vi "LCR_SelectiveWriter.vi"(8 "error in (no error)":errorcluster, 9 "Data Cluster":T3, 10 "Configuration Cluster":T1={"General"={"Config.ini"=path "", "Default Logging Path"=path ""}, "Hardware"={"LCR VISA COM"="", "Measure Rate (1/s)"=0, "Reset on Load?"=FALSE, "Measure Profile"=path ""}, "HM8118 Current Profile"={"Bias Profile"={" Bias Source (OFF)"=0, " Bias Type (Voltage)"=0, "Bias Level (0)"=0.0}, "Measurement Profile"={"Operation Mode (0: Auto)"=0, "Circuit Type (2: Auto)"=2, "Manual Range (1:Range 1 and 25 Ohms)"=1, "Auto Range (T: Enable)"=TRUE}, "Signal Profile"={"Frequency (1kHz)"=1000.0, "Measuring Voltage (1V)"=1.0}, "Integration Profile"={"Averaging (0: Off)"=0, "Averaging Number (2)"=2, "Time (100ms)"=100, "Rate (0: Fast)"=0}, "Trigger Profile"={"Trigger Mode (0: Continuous)"=0}}, "HM8118 New Profile"={"Bias Profile"={" Bias Source (OFF)"=0, " Bias Type (Voltage)"=0, "Bias Level (0)"=0.0}, "Measurement Profile"={"Operation Mode (0: Auto)"=0, "Circuit Type (2: Auto)"=2, "Manual Range (1:Range 1 and 25 Ohms)"=1, "Auto Range (T: Enable)"=TRUE}, "Signal Profile"={"Frequency (1kHz)"=1000.0, "Measuring Voltage (1V)"=1.0}, "Integration Profile"={"Averaging (0: Off)"=0, "Averaging Number (2)"=2, "Time (100ms)"=100, "Rate (0: Fast)"=0}, "Trigger Profile"={"Trigger Mode (0: Continuous)"=0}}, "Operation"={"Operation Mode"=enum."Logging"}} {"HM8118 New Profile"."Trigger Profile"."Trigger Mode (0: Continuous)" items=["Continuous", "Manual", "External"]; "HM8118 New Profile"."Integration Profile"."Rate (0: Fast)" items=["Fast", "Medium", "Slow"]; "HM8118 New Profile"."Integration Profile"."Time (100ms)" min=1 max=999; "HM8118 New Profile"."Integration Profile"."Averaging Number (2)" min=2 max=99; "HM8118 New Profile"."Integration Profile"."Averaging (0: Off)" items=["Off", "Normal", "Averaging"]; "HM8118 New Profile"."Signal Profile"."Measuring Voltage (1V)" min=0.05 max=1.5 step=0.01; "HM8118 New Profile"."Signal Profile"."Frequency (1kHz)" min=20.0 max=200000.0; "HM8118 New Profile"."Measurement Profile"."Manual Range (1:Range 1 and 25 Ohms)" items=["Range 1 and 25 Ohms"=1, "Range 2 and 25 Ohms"=2, "Range 3 and 400 Ohms"=3, "Range 4 and 6.4 kOhms"=4, "Range 5 and 100kOhms"=5, "Range 6 and 100kOhms"=6]; "HM8118 New Profile"."Measurement Profile"."Circuit Type (2: Auto)" items=["Series", "Parallel", "Auto"]; "HM8118 New Profile"."Measurement Profile"."Operation Mode (0: Auto)" items=["Auto", "L+Q", "L+R", "C+D", "C+R", "R+Q", "Z+Theta", "Y+Theta", "R+X", "G+B", "N+Theta", "M"]; "HM8118 New Profile"."Bias Profile"."Bias Type (Voltage)" items=["Voltage", "Current"]; "HM8118 New Profile"."Bias Profile"."Bias Source (OFF)" items=["Off", "Internal", "External"]; "HM8118 Current Profile"."Trigger Profile"."Trigger Mode (0: Continuous)" items=["Continuous", "Manual", "External"]; "HM8118 Current Profile"."Integration Profile"."Rate (0: Fast)" items=["Fast", "Medium", "Slow"]; "HM8118 Current Profile"."Integration Profile"."Time (100ms)" min=1 max=999; "HM8118 Current Profile"."Integration Profile"."Averaging Number (2)" min=2 max=99; "HM8118 Current Profile"."Integration Profile"."Averaging (0: Off)" items=["Off", "Normal", "Averaging"]; "HM8118 Current Profile"."Signal Profile"."Measuring Voltage (1V)" min=0.05 max=1.5 step=0.01; "HM8118 Current Profile"."Signal Profile"."Frequency (1kHz)" min=20.0 max=200000.0; "HM8118 Current Profile"."Measurement Profile"."Manual Range (1:Range 1 and 25 Ohms)" items=["Range 1 and 25 Ohms"=1, "Range 2 and 25 Ohms"=2, "Range 3 and 400 Ohms"=3, "Range 4 and 6.4 kOhms"=4, "Range 5 and 100kOhms"=5, "Range 6 and 100kOhms"=6]; "HM8118 Current Profile"."Measurement Profile"."Circuit Type (2: Auto)" items=["Series", "Parallel", "Auto"]; "HM8118 Current Profile"."Measurement Profile"."Operation Mode (0: Auto)" items=["Auto", "L+Q", "L+R", "C+D", "C+R", "R+Q", "Z+Theta", "Y+Theta", "R+X", "G+B", "N+Theta", "M"]; "HM8118 Current Profile"."Bias Profile"."Bias Type (Voltage)" items=["Voltage", "Current"]; "HM8118 Current Profile"."Bias Profile"."Bias Source (OFF)" items=["Off", "Internal", "External"]}) -> (0 "error out":errorcluster, 2 "Configuration Cluster Out":T1={"General"={"Config.ini"=path "", "Default Logging Path"=path ""}, "Hardware"={"LCR VISA COM"="", "Measure Rate (1/s)"=0, "Reset on Load?"=FALSE, "Measure Profile"=path ""}, "HM8118 Current Profile"={"Bias Profile"={" Bias Source (OFF)"=0, " Bias Type (Voltage)"=0, "Bias Level (0)"=0.0}, "Measurement Profile"={"Operation Mode (0: Auto)"=0, "Circuit Type (2: Auto)"=2, "Manual Range (1:Range 1 and 25 Ohms)"=1, "Auto Range (T: Enable)"=TRUE}, "Signal Profile"={"Frequency (1kHz)"=1000.0, "Measuring Voltage (1V)"=1.0}, "Integration Profile"={"Averaging (0: Off)"=0, "Averaging Number (2)"=2, "Time (100ms)"=100, "Rate (0: Fast)"=0}, "Trigger Profile"={"Trigger Mode (0: Continuous)"=0}}, "HM8118 New Profile"={"Bias Profile"={" Bias Source (OFF)"=0, " Bias Type (Voltage)"=0, "Bias Level (0)"=0.0}, "Measurement Profile"={"Operation Mode (0: Auto)"=0, "Circuit Type (2: Auto)"=2, "Manual Range (1:Range 1 and 25 Ohms)"=1, "Auto Range (T: Enable)"=TRUE}, "Signal Profile"={"Frequency (1kHz)"=1000.0, "Measuring Voltage (1V)"=1.0}, "Integration Profile"={"Averaging (0: Off)"=0, "Averaging Number (2)"=2, "Time (100ms)"=100, "Rate (0: Fast)"=0}, "Trigger Profile"={"Trigger Mode (0: Continuous)"=0}}, "Operation"={"Operation Mode"=enum."Logging"}} {"HM8118 New Profile"."Trigger Profile"."Trigger Mode (0: Continuous)" items=["Continuous", "Manual", "External"]; "HM8118 New Profile"."Integration Profile"."Rate (0: Fast)" items=["Fast", "Medium", "Slow"]; "HM8118 New Profile"."Integration Profile"."Time (100ms)" min=1 max=999; "HM8118 New Profile"."Integration Profile"."Averaging Number (2)" min=2 max=99; "HM8118 New Profile"."Integration Profile"."Averaging (0: Off)" items=["Off", "Normal", "Averaging"]; "HM8118 New Profile"."Signal Profile"."Measuring Voltage (1V)" min=0.05 max=1.5 step=0.01; "HM8118 New Profile"."Signal Profile"."Frequency (1kHz)" min=20.0 max=200000.0; "HM8118 New Profile"."Measurement Profile"."Manual Range (1:Range 1 and 25 Ohms)" items=["Range 1 and 25 Ohms"=1, "Range 2 and 25 Ohms"=2, "Range 3 and 400 Ohms"=3, "Range 4 and 6.4 kOhms"=4, "Range 5 and 100kOhms"=5, "Range 6 and 100kOhms"=6]; "HM8118 New Profile"."Measurement Profile"."Circuit Type (2: Auto)" items=["Series", "Parallel", "Auto"]; "HM8118 New Profile"."Measurement Profile"."Operation Mode (0: Auto)" items=["Auto", "L+Q", "L+R", "C+D", "C+R", "R+Q", "Z+Theta", "Y+Theta", "R+X", "G+B", "N+Theta", "M"]; "HM8118 New Profile"."Bias Profile"."Bias Type (Voltage)" items=["Voltage", "Current"]; "HM8118 New Profile"."Bias Profile"."Bias Source (OFF)" items=["Off", "Internal", "External"]; "HM8118 Current Profile"."Trigger Profile"."Trigger Mode (0: Continuous)" items=["Continuous", "Manual", "External"]; "HM8118 Current Profile"."Integration Profile"."Rate (0: Fast)" items=["Fast", "Medium", "Slow"]; "HM8118 Current Profile"."Integration Profile"."Time (100ms)" min=1 max=999; "HM8118 Current Profile"."Integration Profile"."Averaging Number (2)" min=2 max=99; "HM8118 Current Profile"."Integration Profile"."Averaging (0: Off)" items=["Off", "Normal", "Averaging"]; "HM8118 Current Profile"."Signal Profile"."Measuring Voltage (1V)" min=0.05 max=1.5 step=0.01; "HM8118 Current Profile"."Signal Profile"."Frequency (1kHz)" min=20.0 max=200000.0; "HM8118 Current Profile"."Measurement Profile"."Manual Range (1:Range 1 and 25 Ohms)" items=["Range 1 and 25 Ohms"=1, "Range 2 and 25 Ohms"=2, "Range 3 and 400 Ohms"=3, "Range 4 and 6.4 kOhms"=4, "Range 5 and 100kOhms"=5, "Range 6 and 100kOhms"=6]; "HM8118 Current Profile"."Measurement Profile"."Circuit Type (2: Auto)" items=["Series", "Parallel", "Auto"]; "HM8118 Current Profile"."Measurement Profile"."Operation Mode (0: Auto)" items=["Auto", "L+Q", "L+R", "C+D", "C+R", "R+Q", "Z+Theta", "Y+Theta", "R+X", "G+B", "N+Theta", "M"]; "HM8118 Current Profile"."Bias Profile"."Bias Type (Voltage)" items=["Voltage", "Current"]; "HM8118 Current Profile"."Bias Profile"."Bias Source (OFF)" items=["Off", "Internal", "External"]})   [LabVIEW 2021]
uses:
  Config_Cluster.ctl
  Mode_Enum.ctl
  Data_Cluster.ctl
  Measurement_Cluster.ctl
  LCR_WriteBias.vi
  LCR_WriteConfigMeas.vi
  LCR_WriteSignal.vi
  LCR_WriteIntegration.vi
  LCR_WriteTrigger.vi
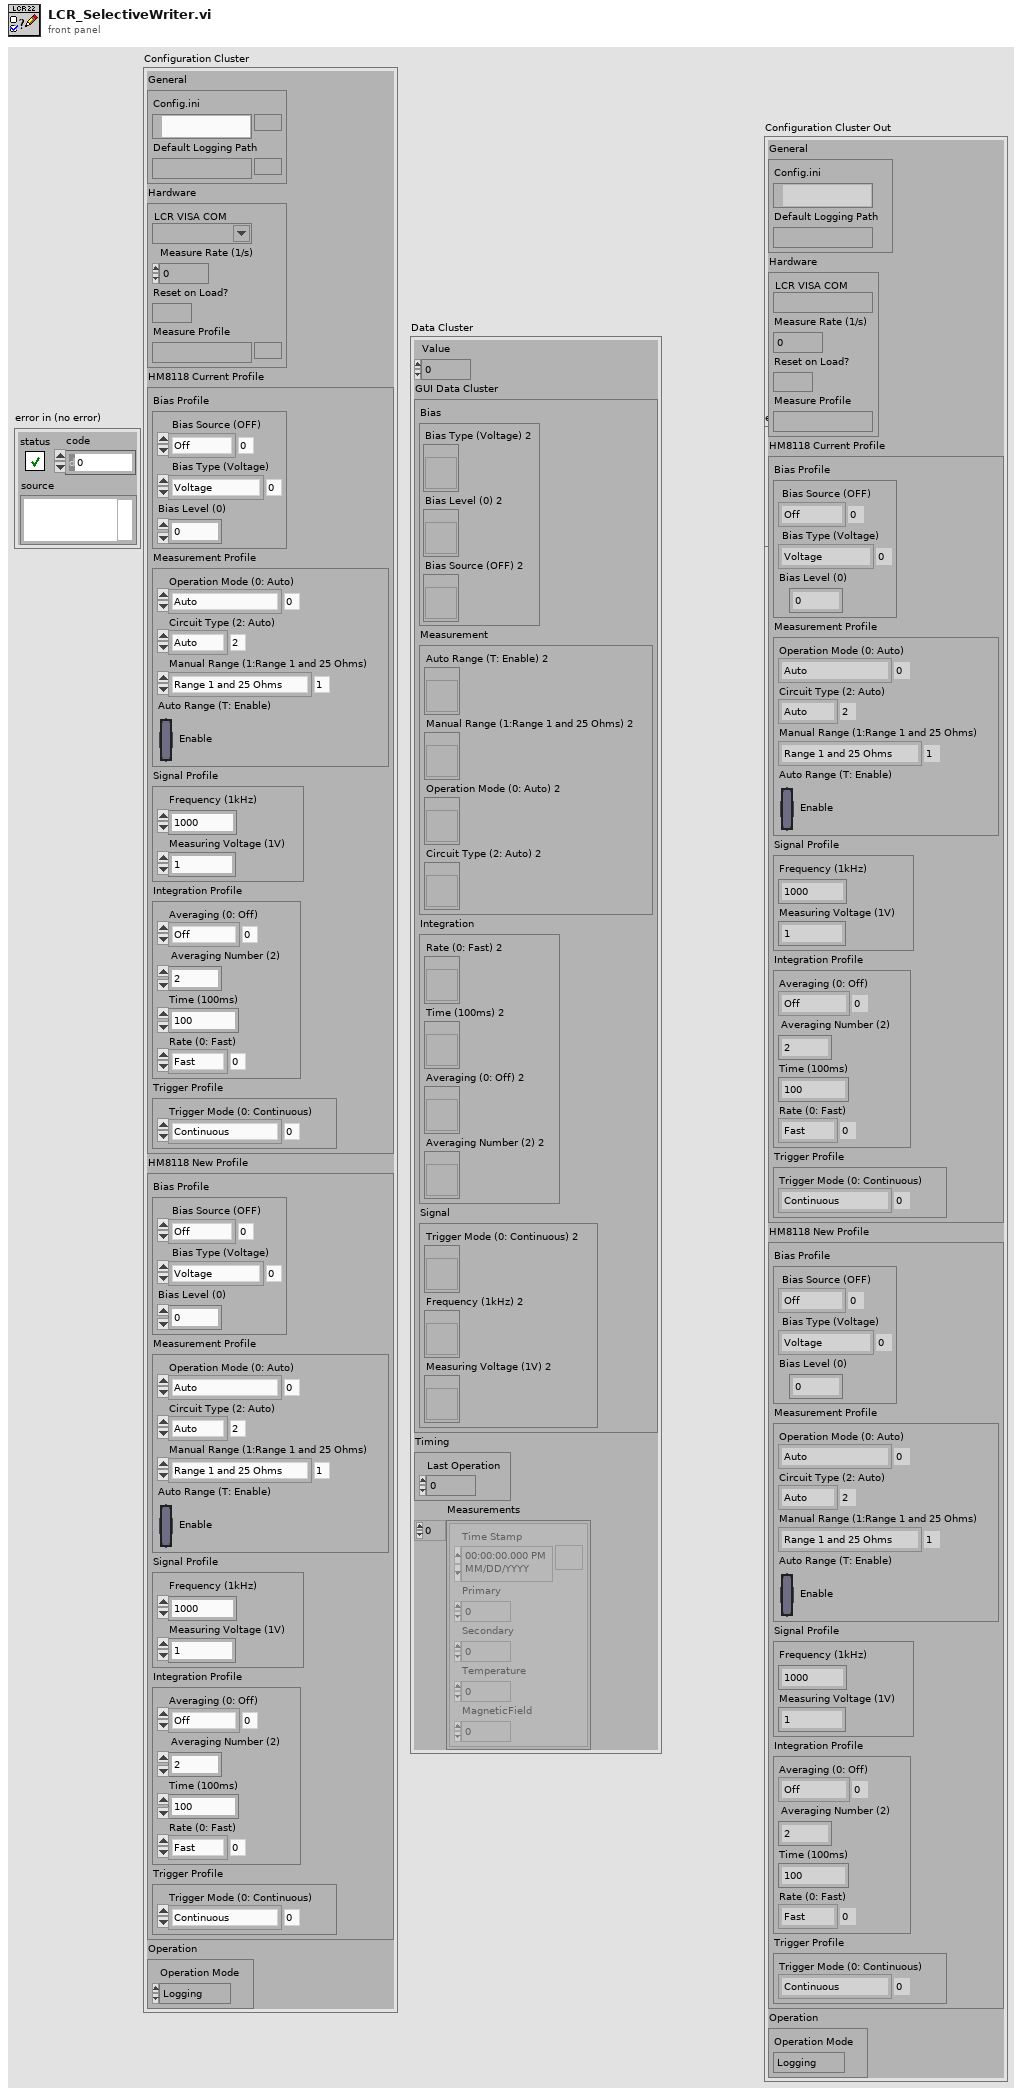
[diagram p1: front panel]
types:
  T1 = typedef "Config_Cluster.ctl" = cluster{"General":cluster{"Config.ini":path, "Default Logging Path":path}, "Hardware":cluster{"LCR VISA COM":refnum<visa-resource-name>, "Measure Rate (1/s)":i32, "Reset on Load?":bool, "Measure Profile":path}, "HM8118 Current Profile":cluster{"Bias Profile":cluster{" Bias Source (OFF)":u8, " Bias Type (Voltage)":u8, "Bias Level (0)":dbl}, "Measurement Profile":cluster{"Operation Mode (0: Auto)":u16, "Circuit Type (2: Auto)":u16, "Manual Range (1:Range 1 and 25 Ohms)":u8, "Auto Range (T: Enable)":bool}, "Signal Profile":cluster{"Frequency (1kHz)":dbl, "Measuring Voltage (1V)":dbl}, "Integration Profile":cluster{"Averaging (0: Off)":u16, "Averaging Number (2)":i32, "Time (100ms)":i32, "Rate (0: Fast)":u16}, "Trigger Profile":cluster{"Trigger Mode (0: Continuous)":u16}}, "HM8118 New Profile":cluster{"Bias Profile":cluster{" Bias Source (OFF)":u8, " Bias Type (Voltage)":u8, "Bias Level (0)":dbl}, "Measurement Profile":cluster{"Operation Mode (0: Auto)":u16, "Circuit Type (2: Auto)":u16, "Manual Range (1:Range 1 and 25 Ohms)":u8, "Auto Range (T: Enable)":bool}, "Signal Profile":cluster{"Frequency (1kHz)":dbl, "Measuring Voltage (1V)":dbl}, "Integration Profile":cluster{"Averaging (0: Off)":u16, "Averaging Number (2)":i32, "Time (100ms)":i32, "Rate (0: Fast)":u16}, "Trigger Profile":cluster{"Trigger Mode (0: Continuous)":u16}}, "Operation":cluster{"Operation Mode":T2}}
  T2 = typedef "Mode_Enum.ctl" = enum16{"Logging", "Idle-Off", "Idle"}
  T3 = typedef "Data_Cluster.ctl" = cluster{"Value":dbl, "GUI Data Cluster":cluster{"Bias":cluster{"Bias Type (Voltage) 2":refnum<vi>, "Bias Level (0) 2":refnum<vi>, "Bias Source (OFF) 2":refnum<vi>}, "Measurement":cluster{"Auto Range (T: Enable) 2":refnum<vi>, "Manual Range (1:Range 1 and 25 Ohms) 2":refnum<vi>, "Operation Mode (0: Auto) 2":refnum<vi>, "Circuit Type (2: Auto) 2":refnum<vi>}, "Integration":cluster{"Rate (0: Fast) 2":refnum<vi>, "Time (100ms) 2":refnum<vi>, "Averaging (0: Off) 2":refnum<vi>, "Averaging Number (2) 2":refnum<vi>}, "Signal":cluster{"Trigger Mode (0: Continuous) 2":refnum<vi>, "Frequency (1kHz) 2":refnum<vi>, "Measuring Voltage (1V) 2":refnum<vi>}}, "Timing":cluster{"Last Operation":dbl}, "Measurements":T4[]}
  T4 = typedef "Measurement_Cluster.ctl" = cluster{"Time Stamp":timestamp, "Primary":dbl, "Secondary":dbl, "Temperature":dbl, "MagneticField":dbl}
  T5 = cluster{"Bias Profile":cluster{" Bias Source (OFF)":u8, " Bias Type (Voltage)":u8, "Bias Level (0)":dbl}, "Measurement Profile":cluster{"Operation Mode (0: Auto)":u16, "Circuit Type (2: Auto)":u16, "Manual Range (1:Range 1 and 25 Ohms)":u8, "Auto Range (T: Enable)":bool}, "Signal Profile":cluster{"Frequency (1kHz)":dbl, "Measuring Voltage (1V)":dbl}, "Integration Profile":cluster{"Averaging (0: Off)":u16, "Averaging Number (2)":i32, "Time (100ms)":i32, "Rate (0: Fast)":u16}, "Trigger Profile":cluster{"Trigger Mode (0: Continuous)":u16}}
  T6 = cluster{" Bias Source (OFF)":u8, " Bias Type (Voltage)":u8, "Bias Level (0)":dbl}
  T7 = cluster{"Operation Mode (0: Auto)":u16, "Circuit Type (2: Auto)":u16, "Manual Range (1:Range 1 and 25 Ohms)":u8, "Auto Range (T: Enable)":bool}
  T8 = cluster{"Frequency (1kHz)":dbl, "Measuring Voltage (1V)":dbl}
  T9 = cluster{"Averaging (0: Off)":u16, "Averaging Number (2)":i32, "Time (100ms)":i32, "Rate (0: Fast)":u16}
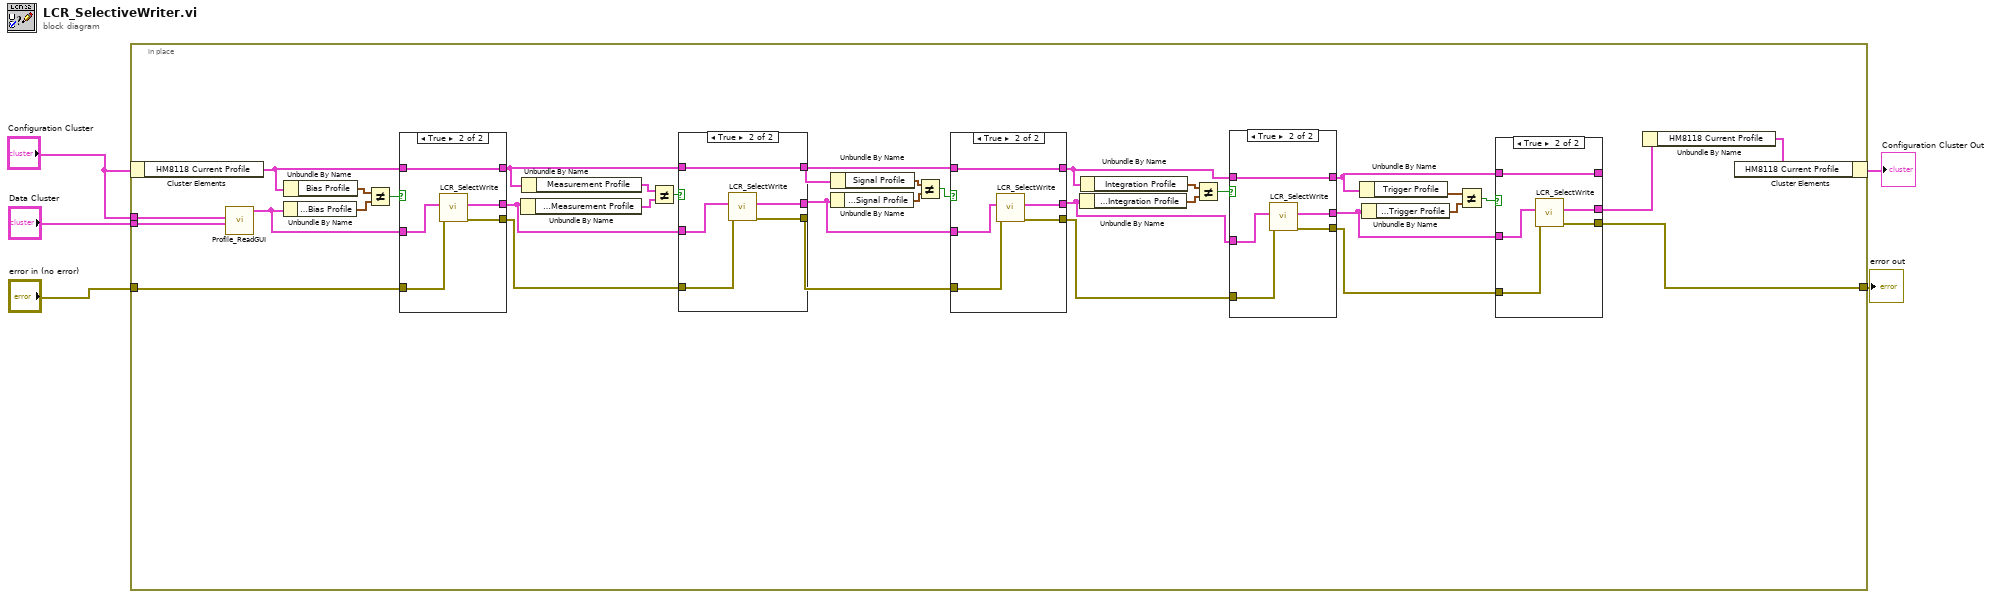
[diagram p0: block diagram]
diagram:
  n1 = in-place {
    in-place-border: "error in (no error)" -> [w39]
    in-place-border: "Data Cluster" -> [w38]
    in-place-border: "Configuration Cluster" -> [w37]
    in-place-border: [w26] -> w2
    n2 = in-place-cluster #1("Configuration Cluster") -> ("HM8118 Current Profile"=w33:T5)
    n3 = call "Profile_ReadGUI.vi"("Data Cluster"=w38, "Configuration Cluster"=w37) -> ("output cluster"=w34:T1)  [unwired: 9 in]
    n4 = Unbundle By Name(w34) -> ("HM8118 Current Profile.Bias Profile"=w35:T6)
    n5 = Unbundle By Name(w33) -> ("Bias Profile"=w36:T6)
    n6 = Not Equal?(x=w36, y=w35) -> (x != y?=w40:bool)
    n7 = case shown="True" w40 {
      tunnel: w39 -> [w73 w80]
      tunnel: w34 -> [w74 w78]
      tunnel: w33 -> [w75 w76]
      tunnel: [w73 w79] -> w30
      tunnel: [w74 w77] -> w21
      tunnel: [w75 w76] -> w25
      frame False {
      }
      frame True {
        n8 = call-poly "LCR_SelectWrite.vi"("error in (no error)"=w80, "Configuration Cluster"=w78) -> ("error out"=w79:errorcluster, "Configuration Cluster Out"=w77:T1)  [unwired: 8 in]
      }
    }
    n9 = Unbundle By Name(w21) -> ("HM8118 Current Profile.Measurement Profile"=w23:T7)
    n10 = Unbundle By Name(w25) -> ("Measurement Profile"=w24:T7)
    n11 = Not Equal?(x=w24, y=w23) -> (x != y?=w22:bool)
    n12 = case shown="True" w22 {
      tunnel: w30 -> [w65 w72]
      tunnel: w21 -> [w66 w70]
      tunnel: w25 -> [w67 w68]
      tunnel: [w65 w71] -> w29
      tunnel: [w66 w69] -> w16
      tunnel: [w67 w68] -> w20
      frame False {
      }
      frame True {
        n13 = call-poly "LCR_SelectWrite.vi"("error in (no error)"=w72, "Configuration Cluster"=w70) -> ("error out"=w71:errorcluster, "Configuration Cluster Out"=w69:T1)  [unwired: 8 in]
      }
    }
    n14 = Unbundle By Name(w16) -> ("HM8118 Current Profile.Signal Profile"=w18:T8)
    n15 = Unbundle By Name(w20) -> ("Signal Profile"=w19:T8)
    n16 = Not Equal?(x=w19, y=w18) -> (x != y?=w17:bool)
    n17 = case shown="True" w17 {
      tunnel: w29 -> [w57 w64]
      tunnel: w16 -> [w58 w62]
      tunnel: w20 -> [w59 w60]
      tunnel: [w57 w63] -> w28
      tunnel: [w58 w61] -> w11
      tunnel: [w59 w60] -> w15
      frame False {
      }
      frame True {
        n18 = call-poly "LCR_SelectWrite.vi"("error in (no error)"=w64, "Configuration Cluster"=w62) -> ("error out"=w63:errorcluster, "Configuration Cluster Out"=w61:T1)  [unwired: 8 in]
      }
    }
    n19 = Unbundle By Name(w11) -> ("HM8118 Current Profile.Integration Profile"=w13:T9)
    n20 = Unbundle By Name(w15) -> ("Integration Profile"=w14:T9)
    n21 = Not Equal?(x=w14, y=w13) -> (x != y?=w12:bool)
    n22 = case shown="True" w12 {
      tunnel: w28 -> [w49 w56]
      tunnel: w11 -> [w50 w54]
      tunnel: w15 -> [w51 w52]
      tunnel: [w49 w55] -> w27
      tunnel: [w50 w53] -> w6
      tunnel: [w51 w52] -> w10
      frame False {
      }
      frame True {
        n23 = call-poly "LCR_SelectWrite.vi"("error in (no error)"=w56, "Configuration Cluster"=w54) -> ("error out"=w55:errorcluster, "Configuration Cluster Out"=w53:T1)  [unwired: 8 in]
      }
    }
    n24 = Unbundle By Name(w10) -> ("Trigger Profile"=w9:cluster{"Trigger Mode (0: Continuous)":u16})
    n25 = Unbundle By Name(w6) -> ("HM8118 Current Profile.Trigger Profile"=w8:cluster{"Trigger Mode (0: Continuous)":u16})
    n26 = Not Equal?(x=w9, y=w8) -> (x != y?=w7:bool)
    n27 = case shown="True" w7 {
      tunnel: w27 -> [w41 w48]
      tunnel: w6 -> [w42 w46]
      tunnel: w10 -> [w43 w44]
      tunnel: [w41 w47] -> w26
      tunnel: [w42 w45] -> w32
      tunnel: [w43 w44] -> _
      frame False {
      }
      frame True {
        n28 = call-poly "LCR_SelectWrite.vi"("error in (no error)"=w48, "Configuration Cluster"=w46) -> ("error out"=w47:errorcluster, "Configuration Cluster Out"=w45:T1)  [unwired: 8 in]
      }
    }
    n29 = Unbundle By Name(w32) -> ("HM8118 Current Profile"=w31:T5)
    n30 = in-place-cluster #1("HM8118 Current Profile"=w31) -> (→"Configuration Cluster Out":T1)
  }
  "error out" <- w2
